vi "fpga_transmission_control_3V6.vi"() -> ()   [LabVIEW 2017]
uses:
  Control 1.ctl
  <vilib>/Instr/_visa.llb/VISA Configure Serial Port (Serial Instr).vi
panel:
  out "Output":bool
  out "outcome":u32
  out "currentType":string
  out "Time":dbl(slide) scale=0.0..100.0
  out "Progress":dbl(slide) scale=0.0..100.0
  in  "error in (no error)":errorcluster
  out "PWM":bool
  out "pattern":u32
  in  "Timeslot":bool
  out "type":string
  out "Kombi Chart":cluster{u16, i16}(graph)
  out "contingency":string
  in  "Array":T2(array[cluster]) {"duration" step=1}
  out "Timeslot":i32
  out "Timer":dbl caption="Elapsed Time (s)"
  out "Sign":bool
  out "deleted portion":u8[](array[numeric])
  out "data":bool
  out "x-y":u16
  out "Error String":string
  out "error out":errorcluster
  out "Timing":u32
  out "Int_pixel":i16
  out "Pixel":u16(graph)
  out "AD_Value":i16
  in  "millisecond timer value 2":u32
  out "AD_Chart":i16(graph)
  in  "Path":path
  out "Read":bool
  in  "Stop Program":bool
  in  "Start":bool
  in  "VISA resource name":refnum<visa-resource-name>
  # "UR Elektronik Biologie\nTerminal V 3.4"
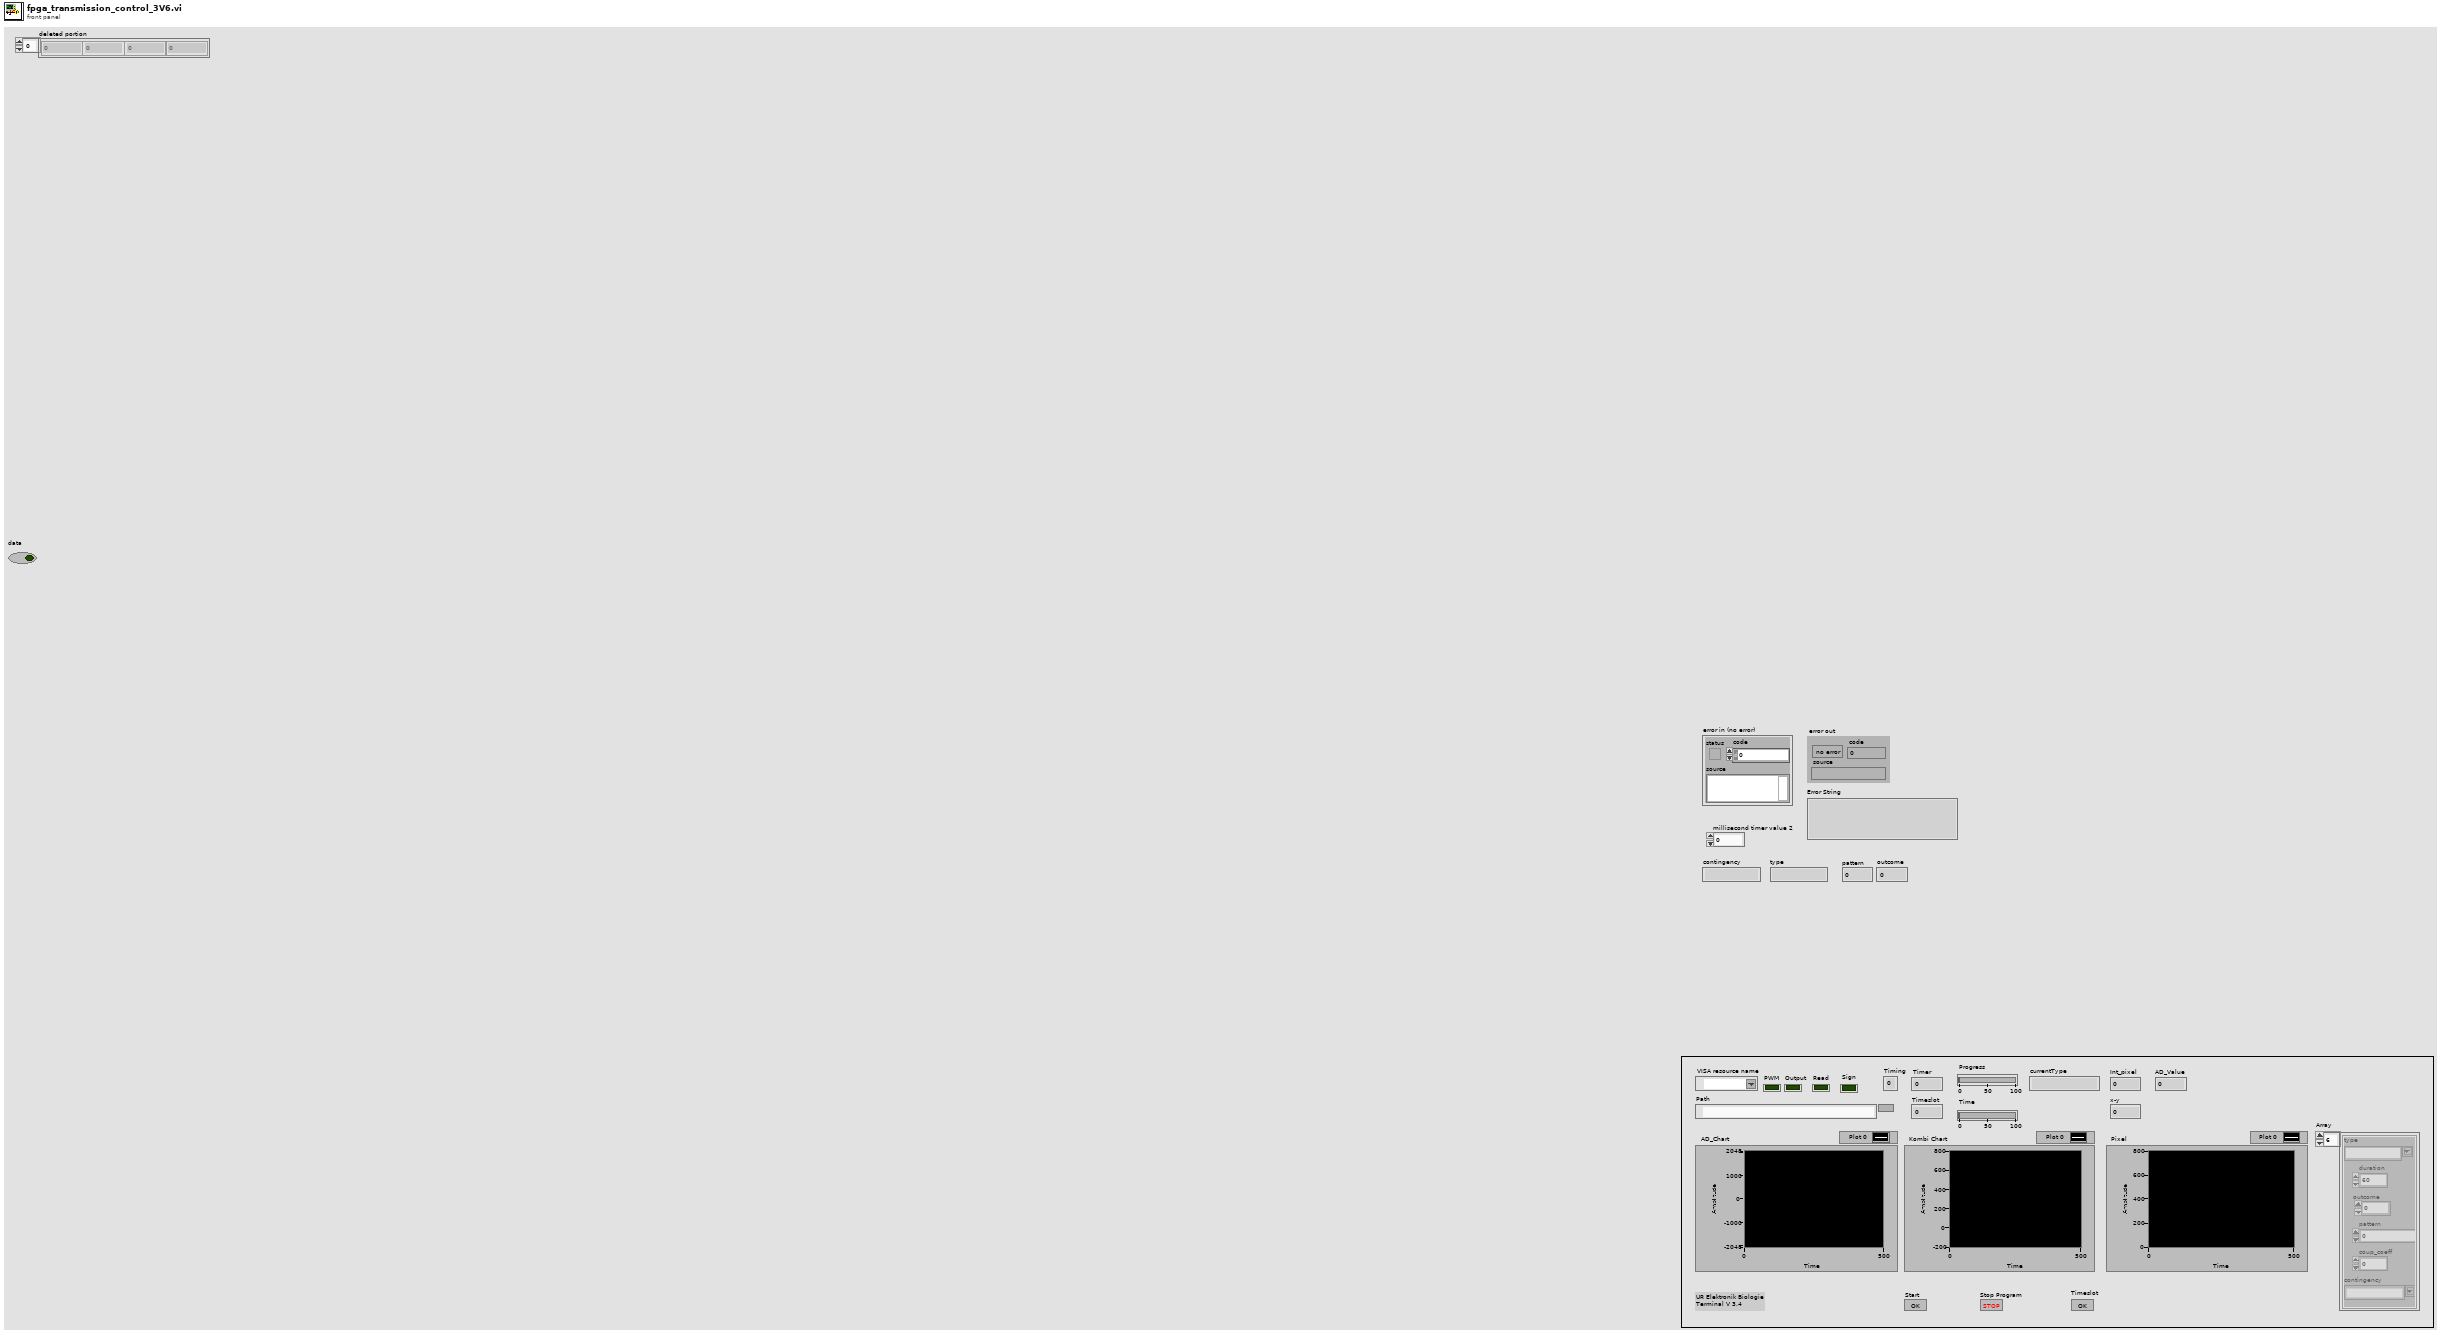
[diagram p1: front panel]
types:
  T1 = typedef "Control 1.ctl" = u32
  T2 = cluster{"type":string, "duration":T1, "outcome":u32, "pattern":u32, "coup_coeff":u32, "contingency":string}[]
  T3 = cluster{"String":string, i32, i32, u32, u32, "String":string}[]
  T4 = enum16{"Idel", "State1", "State2", "State3", "State4"}
  T5 = enum16{"open", "replace", "create", "open or create", "replace or create", "replace or create with confirmation"}
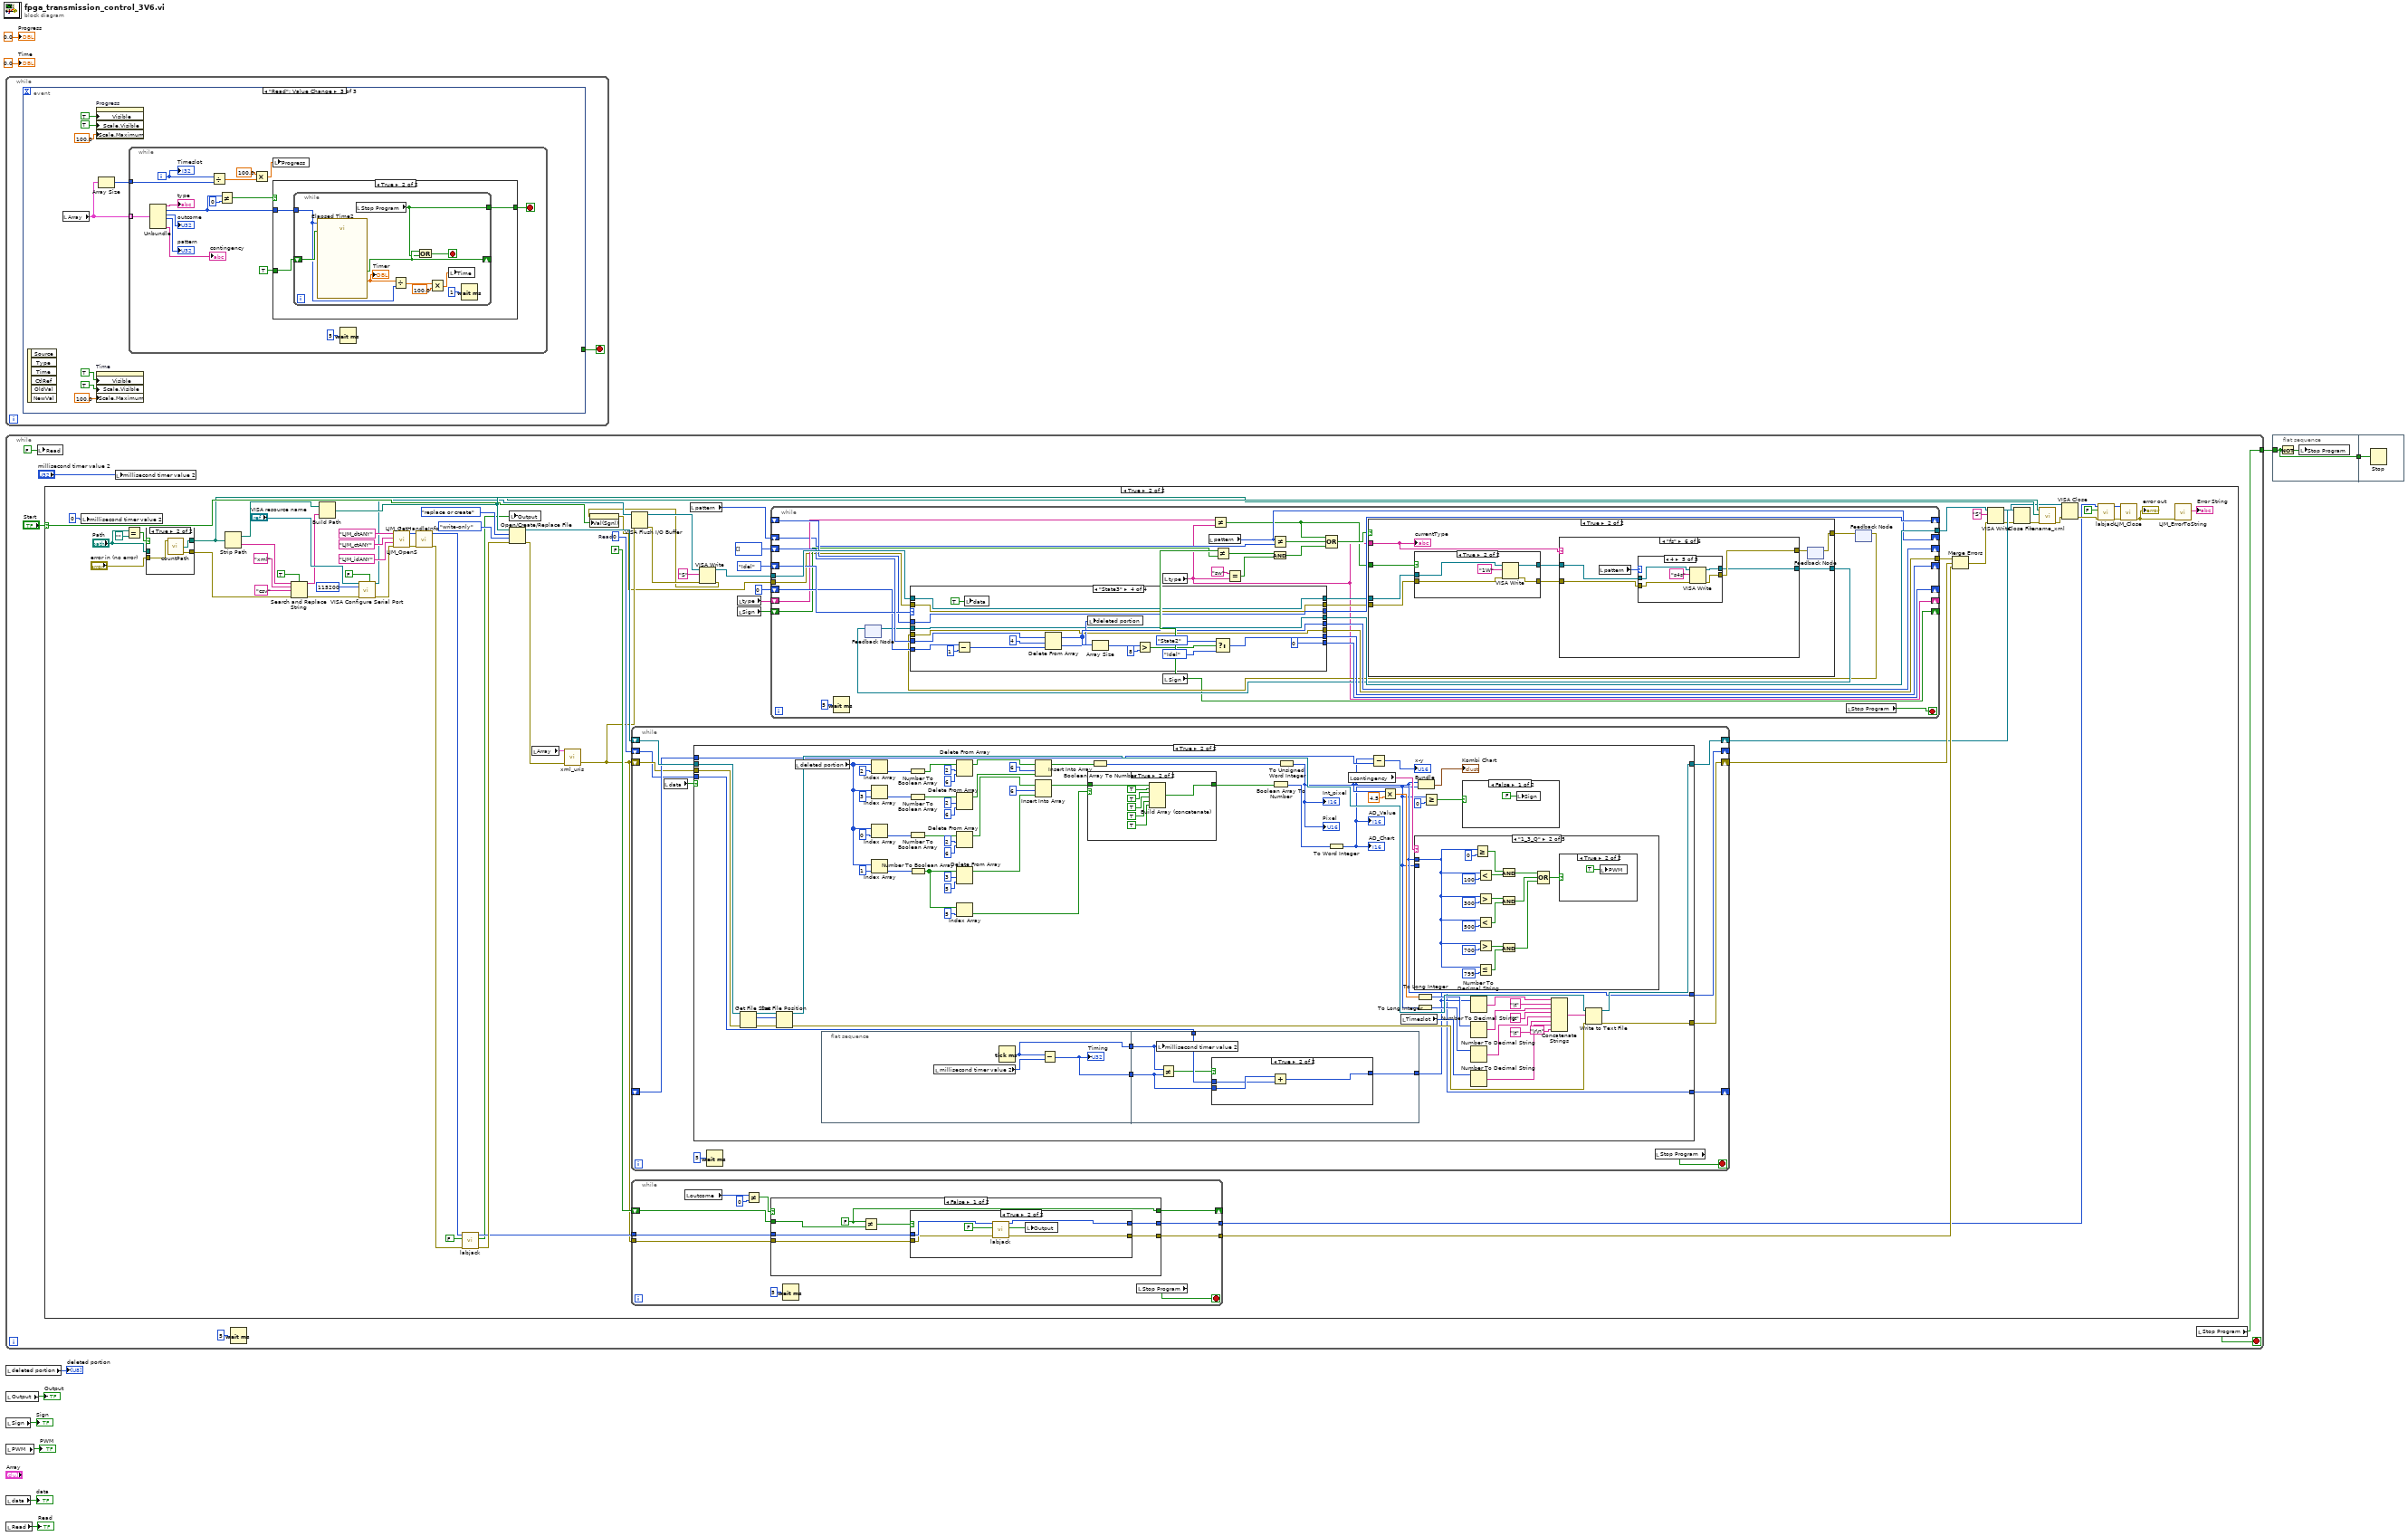
[diagram p0: block diagram]
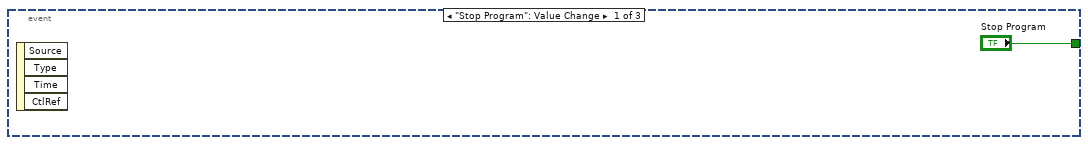
[diagram p2: hidden frame]
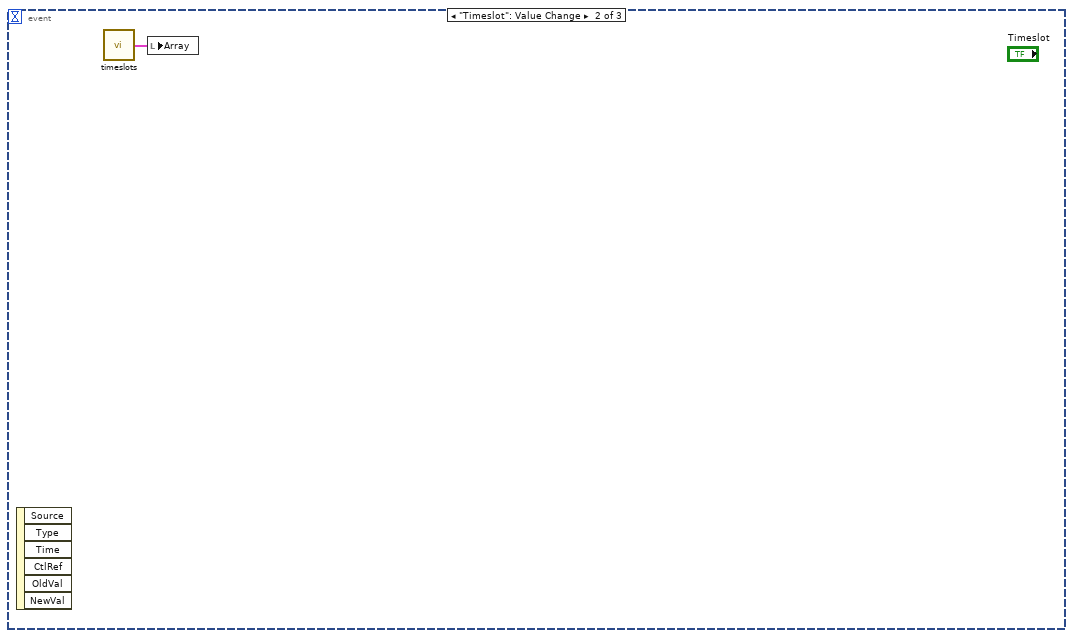
[diagram p3: hidden frame]
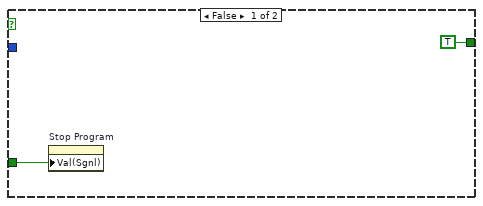
[diagram p4: hidden frame]
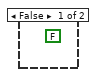
[diagram p5: hidden frame]
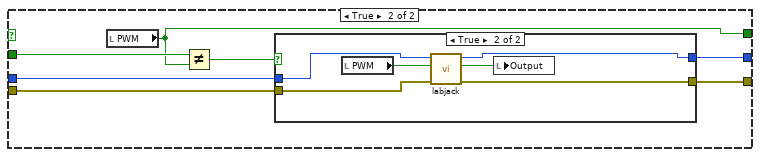
[diagram p8: hidden frame]
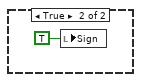
[diagram p11: hidden frame]
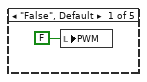
[diagram p12: hidden frame]
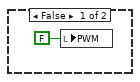
[diagram p13: hidden frame]
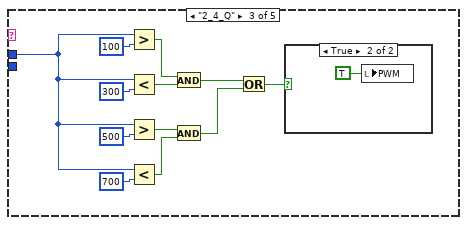
[diagram p14: hidden frame]
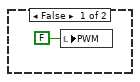
[diagram p15: hidden frame]
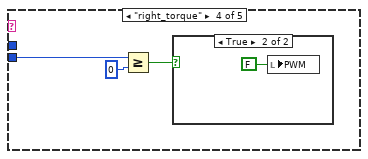
[diagram p16: hidden frame]
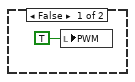
[diagram p17: hidden frame]
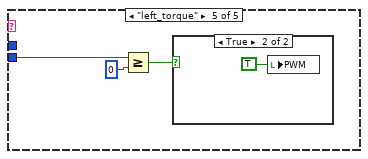
[diagram p18: hidden frame]
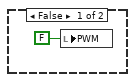
[diagram p19: hidden frame]
diagram:
  n1 = while {
    stop <- w11 stop-if-true
    n2 = event shown="[2] \"Read\": Value Change" {
      selector: _ -> [_ _ _]
      dyn-events: _ -> [_ _ _]
      timeout: _ -> [_ _ _]
      tunnel: ["Stop Program" _ _] -> w11
      event "Stop Program": Value Change {
        n3 = event-data() -> ()  [unwired: 1 in, 4 out]
      }
      event "Timeslot": Value Change {
        n4 = event-data() -> ()  [unwired: 1 in, 6 out]
        n5 = call "timeslots.vi"() -> ("array of clusters"=w13:T3)  [unwired: 2 in]
        n6 = local write "Array"(w13) -> ()
      }
      event "Read": Value Change {
        n7 = event-data() -> ()  [unwired: 1 in, 6 out]
        n8 = local read "Array"() -> (w21:T2)
        n9 = property on="Progress" class="Slide (strict)"("Visible"=TRUE, "Scale.Visible"=TRUE ("Visible"), "Scale.Maximum"=100.0 ("Scale.Range:Maximum")) -> ()  [unwired: 2 in, 2 out]
        n10 = property on="Time" class="Slide (strict)"("Visible"=TRUE, "Scale.Visible"=TRUE ("Visible"), "Scale.Maximum"=100.0 ("Scale.Range:Maximum")) -> ()  [unwired: 2 in, 2 out]
        n11 = Array Size(array=w21) -> (size(s)=w20:i32)
        n12 = while {
          tunnel: w21 -> [w35] mode=indexing
          tunnel: w20 -> [w27]
          i -> [w26]
          stop <- w37 stop-if-true
          n13 = Unbundle(w35) -> ("type"=→"type":string, "duration"=w32:T1, "outcome"=→"outcome":u32, "pattern"=→"pattern":u32, "contingency"=→"contingency":string)  [unwired: 1 out]
          n14 = Divide(x=w26, y=w27) -> (x/y=w25:dbl)
          n15 = Not Equal?(x=w32, y=u32 0) -> (x != y?=w33:bool)
          n16 = Multiply(x=100.0 ("y"), y=w25) -> (x*y=w23:dbl)
          n17 = local write "Progress"(w23) -> ()
          n18 = case shown="True" w33 {
            tunnel: w32 -> [_ w42]
            tunnel: [TRUE w41] -> w37
            tunnel: TRUE -> [w38 w40]
            frame False {
              n19 = property on="Stop Program" class="Bool (strict)"("Val(Sgnl)"=w38) -> ()  [unwired: 2 in, 2 out]
            }
            frame True {
              n20 = while {
                shift-right: [w51] -> _
                shift-left: w40 -> [w52]
                tunnel: [w49] -> w41
                tunnel: w42 -> [w44]
                stop <- w50 stop-if-true
                n21 = call "Elapsed Time2"("Time Target (s)"=w44, "Reset"=w52) -> ("Elapsed Time (s)"=w43:dbl, "Time has Elapsed"=w51:bool)  [unwired: 10 in, 6 out]
                "Timer" <- w43
                n22 = local read "Stop Program"() -> (w49:bool)
                n23 = Divide(x=w43, y=w44) -> (x/y=w47:dbl)
                n24 = Or(x=w51, y=w49) -> (x .or. y?=w50:bool)
                n25 = Multiply(x=w47, y=100.0) -> (x*y=w45:dbl)
                n26 = local write "Time"(w45) -> ()
                n27 = Wait (ms)(milliseconds to wait=u32 1) -> ()  [unwired: 1 out]
              }
            }
          }
          n28 = Wait (ms)(milliseconds to wait=u32 5) -> ()  [unwired: 1 out]
          "Timeslot" <- w26
        }
      }
    }
  }
  n29 = while {
    tunnel: [w56] -> w10
    stop <- w56 stop-if-true
    n30 = local write "Read"(FALSE) -> ()
    n31 = case shown="True" "Start" {
      selector: "Start" -> [_ w120]
      frame False {
        (unwired) FALSE
      }
      frame True {
        n32 = local write "millisecond timer value 2"(u32 0 ("millisecond timer value 2")) -> ()
        n33 = Equal?(x="Path", y=path "") -> (x = y?=w107:bool)
        n34 = case shown="True" w107 {
          tunnel: [w129 w132] -> w72
          tunnel: "Path" -> [w129 _]
          tunnel: [w128 w131] -> w81
          tunnel: "error in (no error)" -> [w128 w130]
          frame False {
          }
          frame True {
            n35 = call "countPath.vi"("error in (no error)"=w130) -> ("error out"=w131:errorcluster, "appended path"=w132:path)
          }
        }
        n36 = Strip Path(path=w72) -> (stripped path=w85:path, name=w84:string)
        n37 = Search and Replace String(case sensitive?=TRUE ("ignore case? (F)"), input string=w84, search string="xml", replace string="csv" ("replace string (\"\")"), error in=w81) -> (result string=w78:string, error out=w80:errorcluster)  [unwired: 3 in, 2 out]
        n38 = Build Path(base path=w85, name or relative path=w78) -> (appended path=w73:path)
        n39 = call-poly "VISA Configure Serial Port"("VISA resource name"="VISA resource name", "Enable Termination\nChar (T)"=FALSE ("Enable Termination\nChar (T)"), "baud rate (9600)"=u32 115200, "error in (no error)"=w80) -> ("VISA resource name out"=w70:refnum<visa-resource-name>, "error out"=w95:errorcluster)  [unwired: 10 in]
        n40 = call "LJM_OpenS.vi"("error in"=w95, "Identifier"="LJM_idANY", "ConnectionType"="LJM_ctANY", "DeviceType"="LJM_dtANY") -> ("error out"=w110:errorcluster, "Handle"=w109:i32)  [unwired: 6 in]
        n41 = call "LJM_GetHandleInfo.vi"("error in"=w110, "Handle In"=w109) -> ("error out"=w112:errorcluster, "Handle Out"=w111:i32)  [unwired: 2 in, 6 out]
        n42 = call "labjack.vi"("error out"=w112, "Boolean"=FALSE, "Handle Out"=w111) -> ("error out 2"=w115:errorcluster, "Boolean 2"=w71:bool, "Handle Out 2"=w114:i32)  [unwired: 6 in]
        n43 = local write "Output"(w71) -> ()
        n44 = Open/Create/Replace File(file path (use dialog)=w73, error in=w115, operation (0:open)=T5."replace or create", access (0:read/write)=enum16{"read/write", "read-only", "write-only"}."write-only") -> (refnum out=w88:refnum<file>, error out=w86:errorcluster)  [unwired: 2 in, 1 out]
        n45 = local read "Array"() -> (w87:T2)
        n46 = call "xml_uris.vi"("error in"=w86, "Array"=w87) -> ("error out"=w60:errorcluster)  [unwired: 2 in, 2 out]
        n47 = VISA Flush I/O Buffer(VISA resource name=w70, error in (no error)=w60) -> (VISA resource name out=w69:refnum<visa-resource-name>, error out=w68:errorcluster)  [unwired: 1 in]
        n48 = while {
          shift-right: [w183] -> w76
          shift-left: w88 -> [w184]
          shift-right: [w179] -> _
          shift-left: _ -> [w182]
          shift-right: [w178] -> w77
          shift-left: w60 -> [w177]
          shift-right: [w176] -> _
          shift-left: u32 0 -> [w175]
          stop <- w181 stop-if-true
          n49 = local read "data"() -> (w180:bool)
          n50 = case shown="True" w180 {
            tunnel: w177 -> [w188 w207]
            tunnel: [w188 w252] -> w178
            tunnel: w184 -> [w187 w213]
            tunnel: [w187 w251] -> w183
            tunnel: [w186 w190] -> w179
            tunnel: w182 -> [w186 w208]
            tunnel: [w185 w194] -> w176
            tunnel: w175 -> [w185 w195]
            frame False {
            }
            frame True {
              n51 = Get File Size(file=w213, error in=w207) -> (refnum out=w257:refnum<file>, size (in bytes)=w256:i64, 0:w255:errorcluster)
              n52 = Set File Position(offset (in bytes) (0)=w256, refnum=w257, error in=w255) -> (refnum out=w253:refnum<file>, error out=w254:errorcluster)  [unwired: 1 in]
              n53 = local read "deleted portion"() -> (w215:u8[])
              n54 = flat-sequence {
                tunnel: [w313] -> w250
                tunnel: [w312] -> w196
                tunnel: w250 -> [w316]
                tunnel: w196 -> [w317]
                tunnel: [w319] -> w194
                tunnel: w195 -> [w318]
                frame #0 {
                  n55 = local read "millisecond timer value 2"() -> (w314:u32)
                  n56 = Tick Count (ms)() -> (millisecond timer value=w313:u32)
                  n57 = Subtract(x=w313, y=w314) -> (x-y=w312:u32)
                  "Timing" <- w312
                }
                frame #1 {
                  n58 = local write "millisecond timer value 2"(w316) -> ()
                  n59 = Not Equal?(x=w316, y=w317) -> (x != y?=w315:bool)
                  n60 = case shown="True" w315 {
                    tunnel: w317 -> [_ w323]
                    tunnel: [u32 0 w322] -> w319
                    tunnel: w318 -> [_ w321]
                    frame False {
                    }
                    frame True {
                      n61 = Add(x=w323, y=w321) -> (x+y=w322:u32)
                    }
                  }
                }
              }
              n62 = Index Array(array=w215, index=2) -> (element=w210:u8)
              n63 = Index Array(array=w215, index=3) -> (element=w209:u8)
              n64 = Index Array(array=w215, index=0) -> (element=w212:u8)
              n65 = Index Array(array=w215, index=1) -> (element=w211:u8)
              n66 = Number To Boolean Array(number=w210) -> (Boolean array=w232:bool[])
              n67 = Number To Boolean Array(number=w209) -> (Boolean array=w235:bool[])
              n68 = Number To Boolean Array(number=w212) -> (Boolean array=w222:bool[])
              n69 = Number To Boolean Array(number=w211) -> (Boolean array=w241:bool[])
              n70 = Delete From Array(array=w232, length=2, index=6 ("length")) -> (array with subset deleted=w245:bool[])  [unwired: 1 out]
              n71 = Delete From Array(array=w235, length=2, index=6) -> (array with subset deleted=w246:bool[])  [unwired: 1 out]
              n72 = Delete From Array(array=w222, length=2, index=6 ("length")) -> (array with subset deleted=w225:bool[])  [unwired: 1 out]
              n73 = Delete From Array(array=w241, length=3, index=5) -> (array with subset deleted=w230:bool[])  [unwired: 1 out]
              n74 = Index Array(array=w241, index=5) -> (element=w243:bool)
              n75 = Insert Into Array(array=w245, index=6, new element=w246) -> (w239:bool[])
              n76 = Insert Into Array(array=w225, index=6, new element=w230) -> (w227:bool[])
              n77 = case shown="True" w243 {
                tunnel: w227 -> [w304 w311]
                tunnel: [w304 w306] -> w244
                frame False {
                }
                frame True {
                  n78 = Build Array (concatenate)(w311, TRUE ("new element/subarray"), TRUE ("new element/subarray"), TRUE ("new element/subarray"), TRUE ("new element/subarray"), TRUE ("element")) -> (w306:bool[])
                }
              }
              n79 = Boolean Array To Number(Boolean array=w239) -> (number=w240:u32)
              n80 = Boolean Array To Number(Boolean array=w244) -> (number=w231:u32)
              n81 = To Unsigned Word Integer(number=w240) -> (unsigned 16bit integer=w190:u16)
              "Pixel" <- w190
              "Int_pixel" <- w190
              n82 = To Word Integer(number=w231) -> (16bit integer=w189:i16)
              "AD_Chart" <- w189
              "AD_Value" <- w189
              n83 = local read "contingency"() -> (w197:string)
              n84 = Subtract(x=w190, y=w208) -> (x-y=→"x-y":u16)
              n85 = Multiply(x=w190, y=4.5) -> (x*y=w199:dbl)
              n86 = local read "Timeslot"() -> (w203:i32)
              n87 = case shown="\"1_3_Q\"" w197 {
                tunnel: w190 -> [_ w262 w288 _ _]
                tunnel: w189 -> [_ _ _ w294 w299]
                frame "False", Default {
                  n88 = local write "PWM"(FALSE ("pwm")) -> ()
                }
                frame "1_3_Q" {
                  n89 = Greater Or Equal?(x=w262, y=u16 0 ("x")) -> (x >= y?=w261:bool)
                  n90 = Less?(x=w262, y=u16 100) -> (x < y?=w272:bool)
                  n91 = Greater?(x=w262, y=u16 300 ("a")) -> (0:w274:bool)
                  n92 = Less?(x=w262, y=u16 500 ("b")) -> (x < y?=w273:bool)
                  n93 = Greater?(x=w262, y=u16 700) -> (0:w271:bool)
                  n94 = Less Or Equal?(x=w262, y=u16 799) -> (x <= y?=w269:bool)
                  n95 = And(x=w261, y=w272) -> (x .and. y?=w267:bool)
                  n96 = And(x=w274, y=w273) -> (x .and. y?=w266:bool)
                  n97 = And(x=w271, y=w269) -> (x .and. y?=w265:bool)
                  n98 = Compound Arithmetic op=OR(w267, w266, w265) -> (w264:bool)
                  n99 = case shown="True" w264 {
                    frame False {
                      n100 = local write "PWM"(FALSE ("pwm")) -> ()
                    }
                    frame True {
                      n101 = local write "PWM"(TRUE ("pwm")) -> ()
                    }
                  }
                }
                frame "2_4_Q" {
                  n102 = Greater?(x=w288, y=u16 100 ("x")) -> (0:w283:bool)
                  n103 = Less?(x=w288, y=u16 300) -> (x < y?=w284:bool)
                  n104 = Greater?(x=w288, y=u16 500 ("a")) -> (0:w287:bool)
                  n105 = Less?(x=w288, y=u16 700 ("b")) -> (x < y?=w285:bool)
                  n106 = And(x=w283, y=w284) -> (x .and. y?=w282:bool)
                  n107 = And(x=w287, y=w285) -> (x .and. y?=w286:bool)
                  n108 = Or(x=w282, y=w286) -> (x .or. y?=w281:bool)
                  n109 = case shown="True" w281 {
                    frame False {
                      n110 = local write "PWM"(FALSE ("pwm")) -> ()
                    }
                    frame True {
                      n111 = local write "PWM"(TRUE ("pwm")) -> ()
                    }
                  }
                }
                frame "right_torque" {
                  n112 = Greater Or Equal?(x=w294, y=i16 0) -> (x >= y?=w295:bool)
                  n113 = case shown="True" w295 {
                    frame False {
                      n114 = local write "PWM"(TRUE ("pwm")) -> ()
                    }
                    frame True {
                      n115 = local write "PWM"(FALSE ("pwm")) -> ()
                    }
                  }
                }
                frame "left_torque" {
                  n116 = Greater Or Equal?(x=w299, y=i16 0) -> (x >= y?=w300:bool)
                  n117 = case shown="True" w300 {
                    frame False {
                      n118 = local write "PWM"(FALSE ("pwm")) -> ()
                    }
                    frame True {
                      n119 = local write "PWM"(TRUE ("pwm")) -> ()
                    }
                  }
                }
              }
              n120 = To Long Integer(number=w199) -> (32bit integer=w198:i32)
              n121 = To Long Integer(number=w189) -> (32bit integer=w201:i32)
              n122 = Bundle(w190, w189) -> (→"Kombi Chart":cluster{u16, i16})  [unwired: 1 in]
              n123 = Greater Or Equal?(x=w189, y=i16 0) -> (x >= y?=w191:bool)
              n124 = case shown="False" w191 {
                frame False {
                  n125 = local write "Sign"(FALSE) -> ()
                }
                frame True {
                  n126 = local write "Sign"(TRUE) -> ()
                }
              }
              n127 = Number To Decimal String(number=w194) -> (decimal integer string=w206:string)  [unwired: 1 in]
              n128 = Number To Decimal String(number=w198) -> (decimal integer string=w247:string)  [unwired: 1 in]
              n129 = Number To Decimal String(number=w201) -> (decimal integer string=w204:string)  [unwired: 1 in]
              n130 = Number To Decimal String(number=w203) -> (decimal integer string=w202:string)  [unwired: 1 in]
              n131 = Concatenate Strings(w206, "\t" ("string"), w247, "\t" ("string"), w204, "\t" ("string"), w202, "\r\n") -> (w214:string)
              n132 = Write to Text File(file (use dialog)=w253, text=w214, error in=w254) -> (refnum out=w251:refnum<file>, error out=w252:errorcluster)  [unwired: 1 in, 1 out]
            }
          }
          n133 = Wait (ms)(milliseconds to wait=u32 5) -> ()  [unwired: 1 out]
          n134 = local read "Stop Program"() -> (w181:bool)
        }
        n135 = while {
          tunnel: w114 -> [w141]
          tunnel: w60 -> [w140]
          shift-right: [w137] -> _
          shift-left: FALSE ("pwm") -> [w143]
          tunnel: [w139] -> w96
          tunnel: [w138] -> w121
          stop <- w142 stop-if-true
          n136 = local read "outcome"() -> (w136:u32)
          n137 = Not Equal?(x=w136, y=u32 0) -> (x != y?=w134:bool)
          n138 = case shown="False" w134 {
            tunnel: w143 -> [w146 w165]
            tunnel: w141 -> [w150 w160]
            tunnel: w140 -> [w148 w161]
            tunnel: [w149 w164] -> w139
            tunnel: [w147 w163] -> w138
            tunnel: [w145 w162] -> w137
            frame False {
              w145 = FALSE ("Boolean")
              n139 = Not Equal?(x=w145, y=w146) -> (x != y?=w144:bool)
              n140 = case shown="True" w144 {
                tunnel: w150 -> [w152 w158]
                tunnel: [w152 w157] -> w149
                tunnel: w148 -> [w151 w156]
                tunnel: [w151 w155] -> w147
                frame False {
                }
                frame True {
                  n141 = call "labjack.vi"("error out"=w156, "Boolean"=FALSE, "Handle Out"=w158) -> ("error out 2"=w155:errorcluster, "Boolean 2"=w153:bool, "Handle Out 2"=w157:i32)  [unwired: 6 in]
                  n142 = local write "Output"(w153) -> ()
                }
              }
            }
            frame True {
              n143 = local read "PWM"() -> (w162:bool)
              n144 = Not Equal?(x=w165, y=w162) -> (x != y?=w159:bool)
              n145 = case shown="True" w159 {
                tunnel: w160 -> [w167 w173]
                tunnel: w161 -> [w166 w172]
                tunnel: [w167 w171] -> w164
                tunnel: [w166 w170] -> w163
                frame False {
                }
                frame True {
                  n146 = local read "PWM"() -> (w169:bool)
                  n147 = call "labjack.vi"("error out"=w172, "Boolean"=w169, "Handle Out"=w173) -> ("error out 2"=w170:errorcluster, "Boolean 2"=w168:bool, "Handle Out 2"=w171:i32)  [unwired: 6 in]
                  n148 = local write "Output"(w168) -> ()
                }
              }
            }
          }
          n149 = Wait (ms)(milliseconds to wait=u32 5) -> ()  [unwired: 1 out]
          n150 = local read "Stop Program"() -> (w142:bool)
        }
        n151 = local read "pattern"() -> (w91:u32)
        n152 = VISA Write(VISA resource name=w69, write buffer="S", error in (no error)=w68) -> (VISA resource name out=w67:refnum<visa-resource-name>, error out=w59:errorcluster)  [unwired: 1 out]
        n153 = property on="Read" class="Bool (strict)"(error in=w59, "Val(Sgnl)"=w120) -> (error out=w58:errorcluster)  [unwired: 1 in, 1 out]
        n154 = local read "type"() -> (w116:string)
        n155 = local read "Sign"() -> (w90:bool)
        n156 = while {
          tunnel: w67 -> [w356]
          tunnel: w58 -> [w324]
          shift-right: [w348] -> _
          shift-left: u8[] [] -> [w355]
          tunnel: [w354] -> w63
          tunnel: [w353] -> w125
          shift-right: [w352] -> _
          shift-left: T4."Idel" -> [w351]
          shift-right: [w350] -> _
          shift-left: _ -> [w349]
          shift-right: [w347] -> _
          shift-left: u8 0 -> [w346]
          shift-right: [w329] -> _
          shift-left: w116 -> [w340]
          shift-right: [w338] -> _
          shift-left: w91 -> [w337]
          shift-right: [w336] -> _
          shift-left: w90 -> [w335]
          stop <- w345 stop-if-true
          n157 = Wait (ms)(milliseconds to wait=u32 5) -> ()  [unwired: 1 out]
          n158 = feedback #1() -> (w343:refnum<visa-resource-name>)  [unwired: 1 in]
          n159 = local read "type"() -> (w329:string)
          n160 = local read "Sign"() -> (w336:bool)
          n161 = local read "pattern"() -> (w338:u32)
          n162 = Not Equal?(x=w340, y=w329) -> (x != y?=w330:bool)
          n163 = Not Equal?(x=w336, y=w335) -> (x != y?=w326:bool)
          n164 = Equal?(x="sw", y=w329) -> (x = y?=w327:bool)
          n165 = Not Equal?(x=w338, y=w337) -> (x != y?=w334:bool)
          n166 = And(x=w326, y=w327) -> (x .and. y?=w325:bool)
          n167 = Compound Arithmetic op=OR(w330, w334, w325) -> (w333:bool)
          n168 = local read "Stop Program"() -> (w345:bool)
          n169 = feedback #2() -> (w341:errorcluster)  [unwired: 1 in]
          n170 = case shown="\"State3\"" w351 {
            tunnel: w356 -> [w472 w491 w511 w529]
            tunnel: w324 -> [w470 w489 w509 w526]
            tunnel: w355 -> [w475 w498 w514 w542]
            tunnel: [w483 w502 w510 w528] -> w354
            tunnel: [w482 w501 w508 w527] -> w353
            tunnel: [w485 w493 w515 w537] -> w352
            tunnel: [w481 w503 w513 w535] -> w350
            tunnel: w349 -> [w480 w504 w513 w535]
            tunnel: [w475 w497 w514 w541] -> w348
            tunnel: [w474 w492 w518 u8 0] -> w347
            tunnel: w346 -> [w474 w492 w516 w533]
            tunnel: [w472 w491 w511 w529] -> w331
            tunnel: w343 -> [w471 w490 w510 w528]
            tunnel: [w470 w489 w509 w526] -> w332
            tunnel: w341 -> [w469 w488 w508 w527]
            frame "Idel", Default {
              n171 = local write "data"(FALSE ("data")) -> ()
              n172 = property class="Serial Instr"(reference=w471, error in=w469) -> (reference out=w483:refnum<visa-resource-name>, error out=w482:errorcluster, "Serial Settings:Number of Bytes at Serial Port"=w481:u32)
              n173 = Equal?(x=w481, y=w480) -> (x = y?=w479:bool)
              n174 = Greater?(x=w481, y=u8 0) -> (0:w478:bool)
              n175 = And(x=w479, y=w478) -> (x .and. y?=w476:bool)
              n176 = Select(t=T4."State1", s=w476, f=T4."Idel") -> (s? t:f=w485:T4)
              n177 = Wait (ms)(milliseconds to wait=u32 5) -> ()  [unwired: 1 out]
            }
            frame "State1" {
              n178 = Array Size(array=w498) -> (size(s)=w500:i32)
              n179 = VISA Read(VISA resource name=w490, byte count=w504, error in (no error)=w488) -> (VISA resource name out=w502:refnum<visa-resource-name>, read buffer=w505:string, return count=w503:u32, error out=w501:errorcluster)
              n180 = String To Byte Array(string=w505) -> (unsigned byte array=w499:u8[])
              n181 = Insert Into Array(array=w498, index=w500, new element=w499) -> (w497:u8[])
              n182 = Array Size(array=w497) -> (size(s)=w495:i32)
              n183 = Greater?(x=w495, y=8) -> (0:w494:bool)
              n184 = Select(t=T4."State2", s=w494, f=T4."State1") -> (s? t:f=w493:T4)
            }
            frame "State2" {
              n185 = Index Array(array=w514, index=w516) -> (element=w522:u8)
              n186 = local write "data"(FALSE) -> ()
              n187 = And(x=w522, y=u8 192) -> (x .and. y?=w523:u8)
              n188 = Equal?(x=u8 0, y=w523) -> (x = y?=w519:bool)
              n189 = Select(t=T4."State3", s=w519, f=T4."State2") -> (s? t:f=w515:T4)
              n190 = Add(x=w516, y=u8 1) -> (x+y=w518:u8)
            }
            frame "State3" {
              n191 = Subtract(x=w533, y=u8 1) -> (x-y=w532:u8)
              n192 = local write "data"(TRUE ("data")) -> ()
              n193 = Delete From Array(array=w542, length=4, index=w532) -> (deleted portion=w534:u8[], array with subset deleted=w541:u8[])
              n194 = local write "deleted portion"(w534) -> ()
              n195 = Array Size(array=w541) -> (size(s)=w540:i32)
              n196 = Greater?(x=w540, y=8) -> (0:w538:bool)
              n197 = Select(t=T4."State2", s=w538, f=T4."Idel") -> (s? t:f=w537:T4)
            }
          }
          n198 = case shown="True" w333 {
            tunnel: w331 -> [w358 w362]
            tunnel: [w358 w365] -> w344
            tunnel: w332 -> [w357 w361]
            tunnel: [w357 w366] -> w342
            tunnel: w329 -> [_ w359]
            tunnel: w330 -> [_ w360]
            frame False {
            }
            frame True {
              n199 = case shown="True" w360 {
                tunnel: [w368 w374] -> w364
                tunnel: [w369 w373] -> w363
                tunnel: w362 -> [w369 w371]
                tunnel: w361 -> [w368 w370]
                frame False {
                }
                frame True {
                  n200 = VISA Write(VISA resource name=w371, write buffer="1W", error in (no error)=w370) -> (VISA resource name out=w373:refnum<visa-resource-name>, error out=w374:errorcluster)  [unwired: 1 out]
                }
              }
              n201 = case shown="\"fs\"" w359 {
                tunnel: w363 -> [w376 w383 w388 w396 w407 w444]
                tunnel: [w378 w382 w387 w390 w406 w443] -> w365
                tunnel: w364 -> [w375 w381 w386 w395 w409 w446]
                tunnel: [w377 w380 w385 w391 w408 w445] -> w367
                frame "False", Default {
                  n202 = VISA Write(VISA resource name=w376, write buffer="s4s", error in (no error)=w375) -> (VISA resource name out=w378:refnum<visa-resource-name>, error out=w377:errorcluster)  [unwired: 1 out]
                }
                frame "optomotorR" {
                  n203 = VISA Write(VISA resource name=w383, write buffer="s3r", error in (no error)=w381) -> (VISA resource name out=w382:refnum<visa-resource-name>, error out=w380:errorcluster)  [unwired: 1 out]
                }
                frame "optomotorL" {
                  n204 = VISA Write(VISA resource name=w388, write buffer="s3l", error in (no error)=w386) -> (VISA resource name out=w387:refnum<visa-resource-name>, error out=w385:errorcluster)  [unwired: 1 out]
                }
                frame "yt" {
                  n205 = local read "pattern"() -> (w394:u32)
                  n206 = VISA Write(VISA resource name=w396, write buffer="s1s", error in (no error)=w395) -> (VISA resource name out=w393:refnum<visa-resource-name>, error out=w392:errorcluster)  [unwired: 1 out]
                  n207 = case shown="9" w394 {
                    tunnel: w393 -> [w399 w403]
                    tunnel: w392 -> [w398 w402]
                    tunnel: [w398 w401] -> w391
                    tunnel: [w399 w400] -> w390
                    frame 0, Default {
                    }
                    frame 9 {
                      n208 = VISA Write(VISA resource name=w403, write buffer="D", error in (no error)=w402) -> (VISA resource name out=w400:refnum<visa-resource-name>, error out=w401:errorcluster)  [unwired: 1 out]
                    }
                  }
                }
                frame "sw" {
                  n209 = local read "pattern"() -> (w405:u32)
                  n210 = case shown="7" w405 {
                    tunnel: w409 -> [w410 w415 w431]
                    tunnel: [w410 w413 w430] -> w408
                    tunnel: w407 -> [w411 w416 w429]
                    tunnel: [w411 w414 w428] -> w406
                    frame 0, Default {
                    }
                    frame 8 {
                      n211 = local read "Sign"() -> (w412:bool)
                      n212 = case shown="False" w412 {
                        tunnel: w415 -> [w418 w425]
                        tunnel: [w417 w424] -> w413
                        tunnel: w416 -> [w420 w423]
                        tunnel: [w419 w422] -> w414
                        frame True {
                          n213 = VISA Write(VISA resource name=w420, write buffer="G", error in (no error)=w418) -> (VISA resource name out=w419:refnum<visa-resource-name>, error out=w417:errorcluster)  [unwired: 1 out]
                        }
                        frame False {
                          n214 = VISA Write(VISA resource name=w423, write buffer="B", error in (no error)=w425) -> (VISA resource name out=w422:refnum<visa-resource-name>, error out=w424:errorcluster)  [unwired: 1 out]
                        }
                      }
                    }
                    frame 7 {
                      n215 = local read "Sign"() -> (w427:bool)
                      n216 = case shown="True" w427 {
                        tunnel: w431 -> [w433 w440]
                        tunnel: [w432 w439] -> w430
                        tunnel: w429 -> [w435 w438]
                        tunnel: [w434 w437] -> w428
                        frame False {
                          n217 = VISA Write(VISA resource name=w435, write buffer="G", error in (no error)=w433) -> (VISA resource name out=w434:refnum<visa-resource-name>, error out=w432:errorcluster)  [unwired: 1 out]
                        }
                        frame True {
                          n218 = VISA Write(VISA resource name=w438, write buffer="B", error in (no error)=w440) -> (VISA resource name out=w437:refnum<visa-resource-name>, error out=w439:errorcluster)  [unwired: 1 out]
                        }
                      }
                    }
                  }
                }
                frame "fs" {
                  n219 = local read "pattern"() -> (w442:u32)
                  n220 = case shown="4" w442 {
                    tunnel: w446 -> [w447 w453 w458 w463 w468]
                    tunnel: [w447 w451 w456 w461 w466] -> w445
                    tunnel: w444 -> [w448 w452 w457 w462 w467]
                    tunnel: [w448 w450 w455 w460 w465] -> w443
                    frame 0, Default {
                    }
                    frame 3 {
                      n221 = VISA Write(VISA resource name=w452, write buffer="s3s", error in (no error)=w453) -> (VISA resource name out=w450:refnum<visa-resource-name>, error out=w451:errorcluster)  [unwired: 1 out]
                    }
                    frame 2 {
                      n222 = VISA Write(VISA resource name=w457, write buffer="s2s", error in (no error)=w458) -> (VISA resource name out=w455:refnum<visa-resource-name>, error out=w456:errorcluster)  [unwired: 1 out]
                    }
                    frame 1 {
                      n223 = VISA Write(VISA resource name=w462, write buffer="s1s", error in (no error)=w463) -> (VISA resource name out=w460:refnum<visa-resource-name>, error out=w461:errorcluster)  [unwired: 1 out]
                    }
                    frame 4 {
                      n224 = VISA Write(VISA resource name=w467, write buffer="s4s", error in (no error)=w468) -> (VISA resource name out=w465:refnum<visa-resource-name>, error out=w466:errorcluster)  [unwired: 1 out]
                    }
                  }
                }
              }
              n225 = feedback #3() -> (w366:errorcluster)  [unwired: 1 in]
              n226 = feedback-in #3(w367) -> ()
              "currentType" <- w359
            }
          }
          n227 = feedback-in #1(w344) -> ()
          n228 = feedback-in #2(w342) -> ()
        }
        n229 = Merge Errors(w125, w77, w121) -> (w65:errorcluster)
        n230 = VISA Write(VISA resource name=w63, write buffer="S", error in (no error)=w65) -> (VISA resource name out=w62:refnum<visa-resource-name>, error out=w64:errorcluster)  [unwired: 1 out]
        n231 = Close File(refnum=w76, error in=w64) -> (error out=w75:errorcluster)  [unwired: 1 out]
        n232 = call "rename_xml.vi"("error in"=w75, "xml"=w72, "csv"=w73) -> ("error out"=w74:errorcluster)  [unwired: 4 in]
        n233 = VISA Close(VISA resource name=w62, error in (no error)=w74) -> (error out=w101:errorcluster)
        n234 = call "labjack.vi"("error out"=w101, "Boolean"=FALSE, "Handle Out"=w96) -> ("error out 2"=w102:errorcluster, "Handle Out 2"=w100:i32)  [unwired: 6 in, 1 out]
        n235 = call "LJM_Close.vi"("error in"=w102, "Handle"=w100) -> ("error out"=w99:errorcluster)  [unwired: 9 in]
        "error out" <- w99
        n236 = call "LJM_ErrorToString.vi"("error in"=w99) -> ("String"=→"Error String":string)  [unwired: 10 in]
      }
    }
    n237 = local write "millisecond timer value 2"("millisecond timer value 2") -> ()
    n238 = Wait (ms)(milliseconds to wait=u32 5) -> ()  [unwired: 1 out]
    n239 = local read "Stop Program"() -> (w56:bool)
  }
  n240 = local read "deleted portion"() -> (→"deleted portion":u8[])
  n241 = local read "Output"() -> (→"Output":bool)
  n242 = local read "Sign"() -> (→"Sign":bool)
  n243 = local read "PWM"() -> (→"PWM":bool)
  n244 = local read "data"() -> (→"data":bool)
  n245 = local read "Read"() -> (→"Read":bool)
  n246 = flat-sequence {
    tunnel: w10 -> [w547]
    tunnel: [w547] -> w9
    tunnel: w9 -> [w548]
    frame #0 {
      n247 = Not(x=w547) -> (.not. x?=w546:bool)
      n248 = local write "Stop Program"(w546) -> ()
    }
    frame #1 {
      n249 = Stop(stop? (T)=w548) -> ()
    }
  }
  "Progress" <- 0.0 ("Slide")
  "Time" <- 0.0 ("Progress 2")
